vi "ActionVIOnDelete.vi"(6 "All deleted Refs":T1[](array[typedef]) format="%.0x", 8 "error in (no error)":errorcluster, 11 "Item Ref in":T1 format="%.0x") -> (0 "error out":errorcluster, 3 "Item Ref out":T1 format="%.0x")   [LabVIEW 2019, in "Control Addon System Explorer.lvlib"]
uses:
  Control Addon System Explorer.lvlib
  <vilib>/NI VeriStand/Custom Device API/Custom Device Item Ref.ctl
  <vilib>/NI VeriStand/Custom Device API/Custom Device API.lvlib
  Shared/Control Addon Shared.lvlib
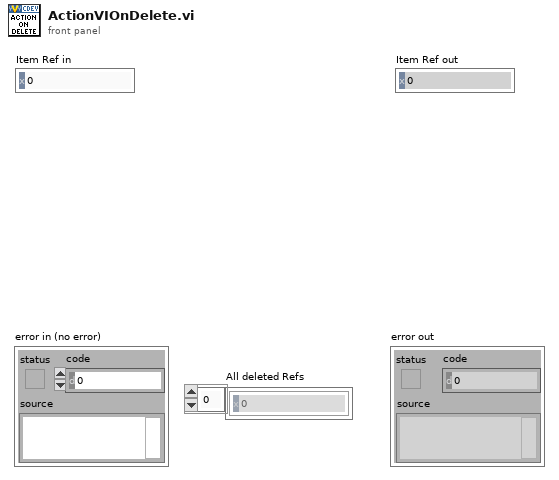
[diagram p1: front panel]
types:
  T1 = typedef "Custom Device API.lvlib/Custom Device Item Ref.ctl" = u64
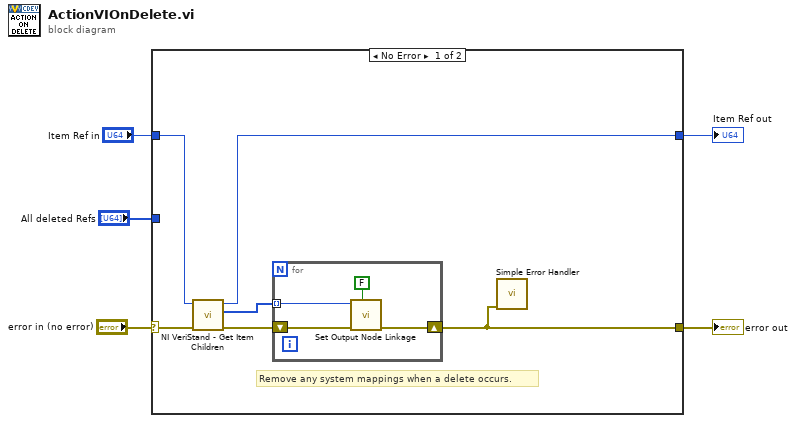
[diagram p0: block diagram]
diagram:
  n1 = case shown="No Error" "error in (no error)" {
    selector: "error in (no error)" -> [w10 w17]
    tunnel: [w11 w17] -> w4
    tunnel: "Item Ref in" -> [w8 w16]
    tunnel: [w7 w16] -> w2
    tunnel: "All deleted Refs" -> [_ _]
    frame No Error {
      # "Remove any system mappings when a delete occurs."
      n2 = call <vilib>:"NI VeriStand - Get Item Children.vi"("error in (no error)"=w10, "Item Ref in"=w8) -> ("error out"=w9:errorcluster, "Child Refs"=w6:T1[], "Item Ref out"=w7:T1)  [unwired: 6 in, 1 out]
      n3 = for {
        shift-right: [w13] -> w11
        shift-left: w9 -> [w14]
        tunnel: w6 -> [w12] mode=indexing
        n4 = call "Set Output Node Linkage.vi"("Add?"=FALSE ("Add? (T)"), "error in"=w14, "Section Ref in"=w12) -> ("error out"=w13:errorcluster)  [unwired: 7 in, 1 out]
      }
      n5 = call <vilib>:"Simple Error Handler.vi"("error in (no error)"=w11) -> ()  [unwired: 4 in, 5 out]
    }
    frame Error {
    }
  }
  "error out" <- w4
  "Item Ref out" <- w2
